vi "crio_RT_Radial_Antagonist_Closed_Loop_Vibration_Injection_with_Data_Logging.vi"() -> ()   [LabVIEW 2019]
uses:
  <vilib>/LabVIEW Targets/FPGA/cRIO/shared/nicrio_ModuleControls/nicrio_cRIO-9237_ExcitationVoltageRing.ctl
  <vilib>/Platform/TimedLoop/XDataNode/timing_clust.ctl
  <vilib>/Platform/TimedLoop/XDataNode/nitl_modes.ctl
  <vilib>/Platform/TimedLoop/XDataNode/wakeup.ctl
  <vilib>/FPGAPlugInAG/cRIO-9074/niLvFpga_Open_cRIO-9074.vi
  <vilib>/rvi/interface/common/dynamic/niFpgaDynamicAddResources.vi
  <vilib>/Utility/file.llb/Write Delimited Spreadsheet (string).vi
  <vilib>/Utility/error.llb/Error Cluster From Error Code.vi
  <vilib>/rvi/errors/niLvFpgaAdjustHostInterfaceError.vi
  <vilib>/Utility/file.llb/Write Delimited Spreadsheet (DBL).vi
  <vilib>/FPGAPlugInAG/Dynamic/niLvFpga_Close_Dynamic.vi
  <vilib>/rvi/interface/nirviOpenFPGA/nirviOpenFPGA.xnode
  On Call Bitfiles/gpass2_FPGATarget2_crioFPGAAntagoni_uWzRZvtrb5U.lvbitx
  <vilib>/rvi/interface/nirviReadWriteControl/nirviReadWriteControl.xnode
  <vilib>/platform/TimedLoop/XDataNode/XDataNode.xnode
  <vilib>/rvi/interface/nirviCloseFPGA/nirviCloseFPGA.xnode
  NiFpgaLv.dll
  <vilib>/rvi/interface/Simulation/niFpgaSimulationCallBeginRW.vi
  <vilib>/Platform/TimedLoop/XDataNode/XDNodeRunTimeDep.lvlib
panel:
  in  "LAC Gain Scaler":T1={"proportional gain"=100.0, "integral gain"=100000000.0}
  out "Trajectory time":dbl
  out "start time":timestamp
  out "LabVIEW TimeStamp":timestamp
  out "VCA Measured Position":i32=4
  out "LAC Setpoint":i32
  out "Rail Setpoint":i16
  out "VCA Setpoint":i32
  out "appended array":i32[](array[numeric])
  in  "Channel Names":string[](array[string])=["Channel 1", "Channel 2", "Channel 3", "Channel 4", "Channel 5"]
  in  "Header Info":string[][](array[string])=[["Test Name", "Operator", "UUT"], ["Voltage", "National Instruments", "AA123"]]
  out "error out":errorcluster
  out "log file path":path
  in  "precision test .csv name":string="precision_test.csv"
  in  "Default sin gain":dbl=20.0
  out "rail Platform Position":i16=4000
  out "LAC Measured Position":i32
  in  "VCA Loop Period(us)":i64=2000
  in  "VCA Position Reset":bool
  in  "VCA Velocity Interval (uSec)":u32=1000
  in  "LAC Position Reset":bool
  in  "LAC Velocity Interval (uSec)":u32=1000
  in  "LAC Lock":bool
  in  "Rail Manual Operation":bool
  in  "Rail Stepper Enable":bool
  in  "Rail Stepper Direction":bool
  in  "Half Peirod (pulse 40MHz)":u32=10000
  out "LAC Actual Gain":T1={"proportional gain"=0.009545455, "integral gain"=1.2626262e-09}
  in  "LAC manual control":T2={"manual? (F)"=FALSE, "manual input (0)"=-0.83838385} {"manual input (0)" scale=-1.0..1.0}
  in  "LAC setpoint":i32(slide)=2700 scale=0.0..4500.0
  in  "LAC Gains":T1={"proportional gain"=0.95454544, "integral gain"=0.64646465} {"proportional gain" scale=0.0..1.0; "integral gain" scale=0.0..1.0}
  in  "Rail Desired Position":i16(slide)=4000 scale=0.0..20000.0
  in  "PWM Frequency (default 20kHz)":i32=20000
  in  "Excitation Voltage":T3 items=["2.5 Volts", "3.3 Volts", "5.0 Volts", "10.0 Volts", "External Excitation"]
  out "scaled load cell reading":fxp<+/-,24,24>
  in  "VCA Manual Control":T2
  in  "VCA Gains":T1={"proportional gain"=0.25, "integral gain"=0.7979798} {"proportional gain" scale=0.0..1.0; "integral gain" scale=0.0..1.0}
  out "VCA Actual Gain":T1={"proportional gain"=0.0009797979, "integral gain"=7.979798e-09}
  in  "VCA Gain Scaler":T1={"proportional gain"=1000.0, "integral gain"=100000000.0}
  out "VCA Force Setpoint":sgl
  out "VCA Force":dbl(graph)
  out "PWM":sgl(graph)=0.061072454
  out "ControllerPWM Output":sgl=0.061072454
  out "ms to next point":u32=50500
  in  "Start Fequency":dbl=0.2
  out "Current Sweeping frequency":dbl=0.2
  in  "End Frequency":i32=20
  in  "Frequency Increment":dbl=1.0
  in  "Start Sweep":bool
  in  "Frequency":dbl=0.2
  in  "Lock_loop_rate":u32=5000
  in  "sin_gain":fxp<+,32,10>=0.25
  in  "sin_offset":fxp<+/-,32,10>=0.5
  in  "stop":bool
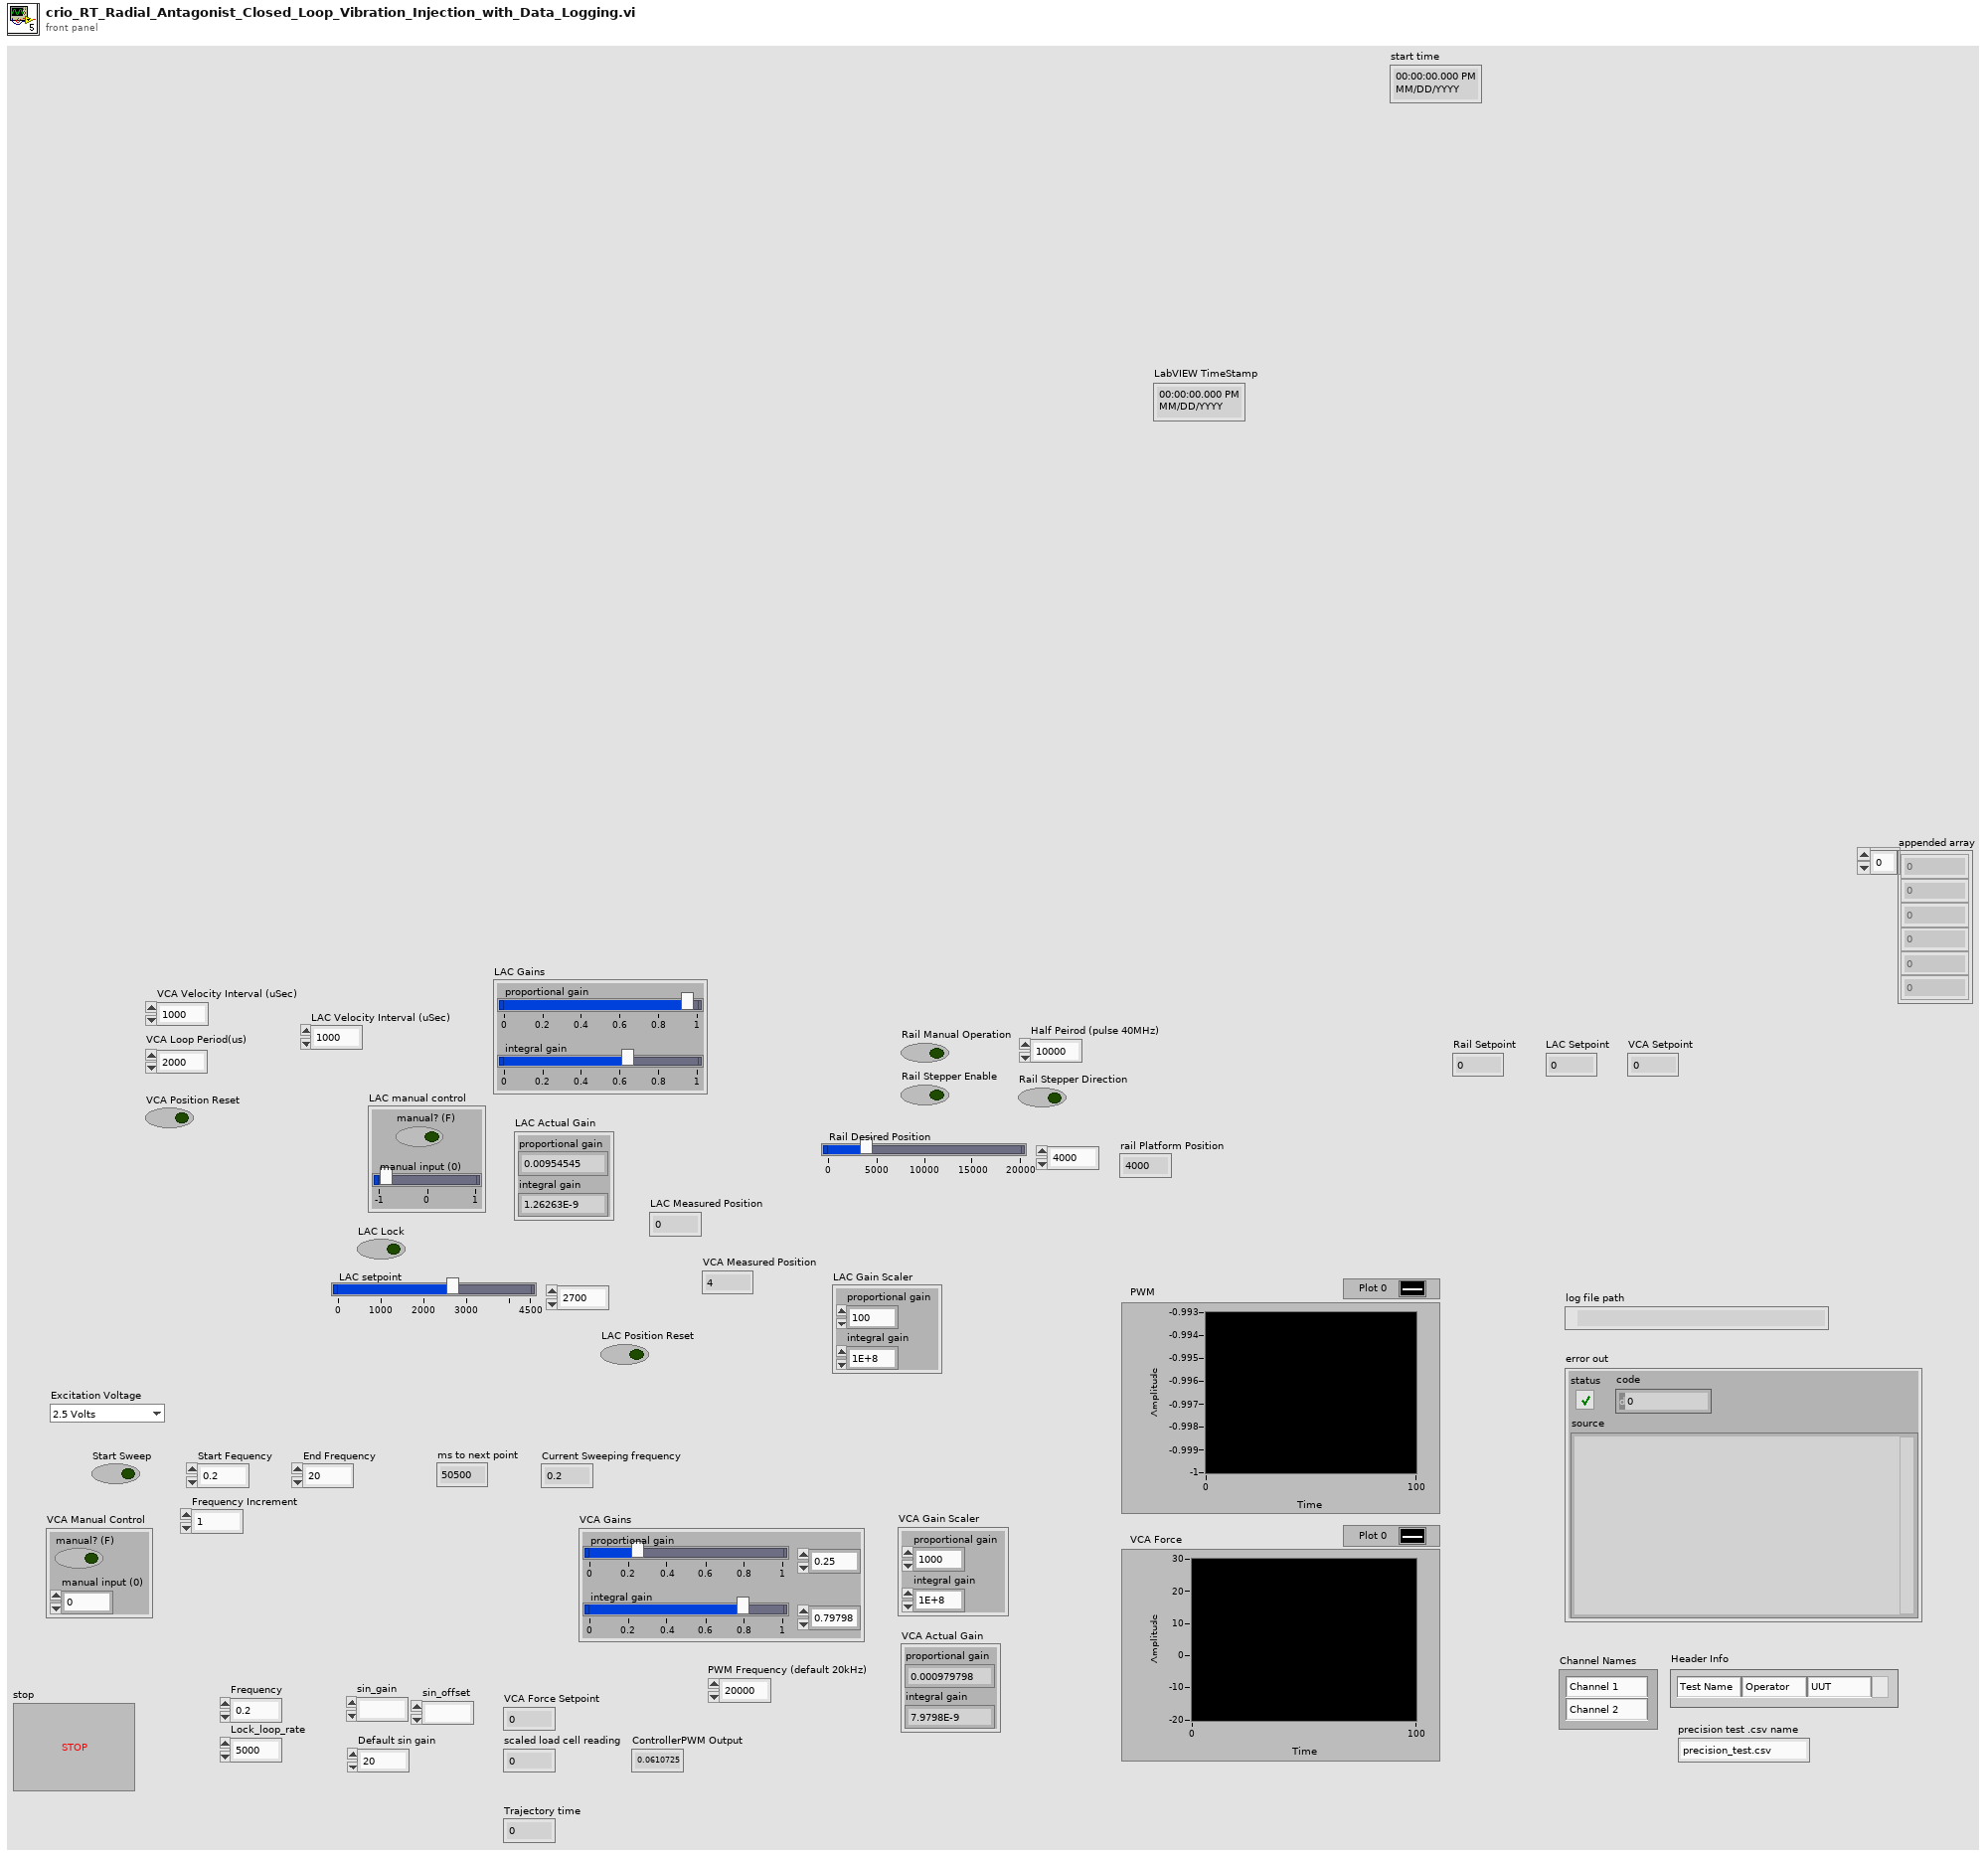
[diagram p1: front panel]
types:
  T1 = cluster{"proportional gain":sgl, "integral gain":sgl}
  T2 = cluster{"manual? (F)":bool, "manual input (0)":sgl}
  T3 = typedef "nicrio_cRIO-9237_ExcitationVoltageRing.ctl" = u8
  T4 = typedef "XDNodeRunTimeDep.lvlib/timing_clust.ctl" = cluster{"Expected End [f-1]":u64, "Actual End [f-1]":u64, "Finished Late? [f-1]":bool, "Expected End [i-1]":u64, "Actual End [i-1]":u64, "Finished Late? [i-1]":bool, "Expected Start [i]":u64, "Actual Start [i]":u64, "Expected Start [f]":u64, "Actual Start [f]":u64, "Source Name":string, "Structure Name":string, "Period":i64, "Deadline":i64, "Offset":i64, "Start":i64, "Priority":i32, "Timeout":i32, "Mode":T5, "Wakeup Reason":T6, "Error":errorcluster, "Source Type":string, "Secondary Source Type":string, "Global End Time":u64, "Global Start Time":u64, "Frame Duration":u64, "Iteration Duration":u64, "Assigned CPU":i32, "I/O Scan Engine Mode":u32}
  T5 = typedef "XDNodeRunTimeDep.lvlib/nitl_modes.ctl" = enum32{"No Change", "Process missed periods, maintain original phase", "Discard missed periods, maintain original phase", "Process missed periods, ignore original phase", "Discard missed periods, ignore original phase"}
  T6 = typedef "XDNodeRunTimeDep.lvlib/wakeup.ctl" = enum32{"Normal", "Aborted", "Asynchronous wakeup", "Timing source error", "Timed loop error", "Timeout"}
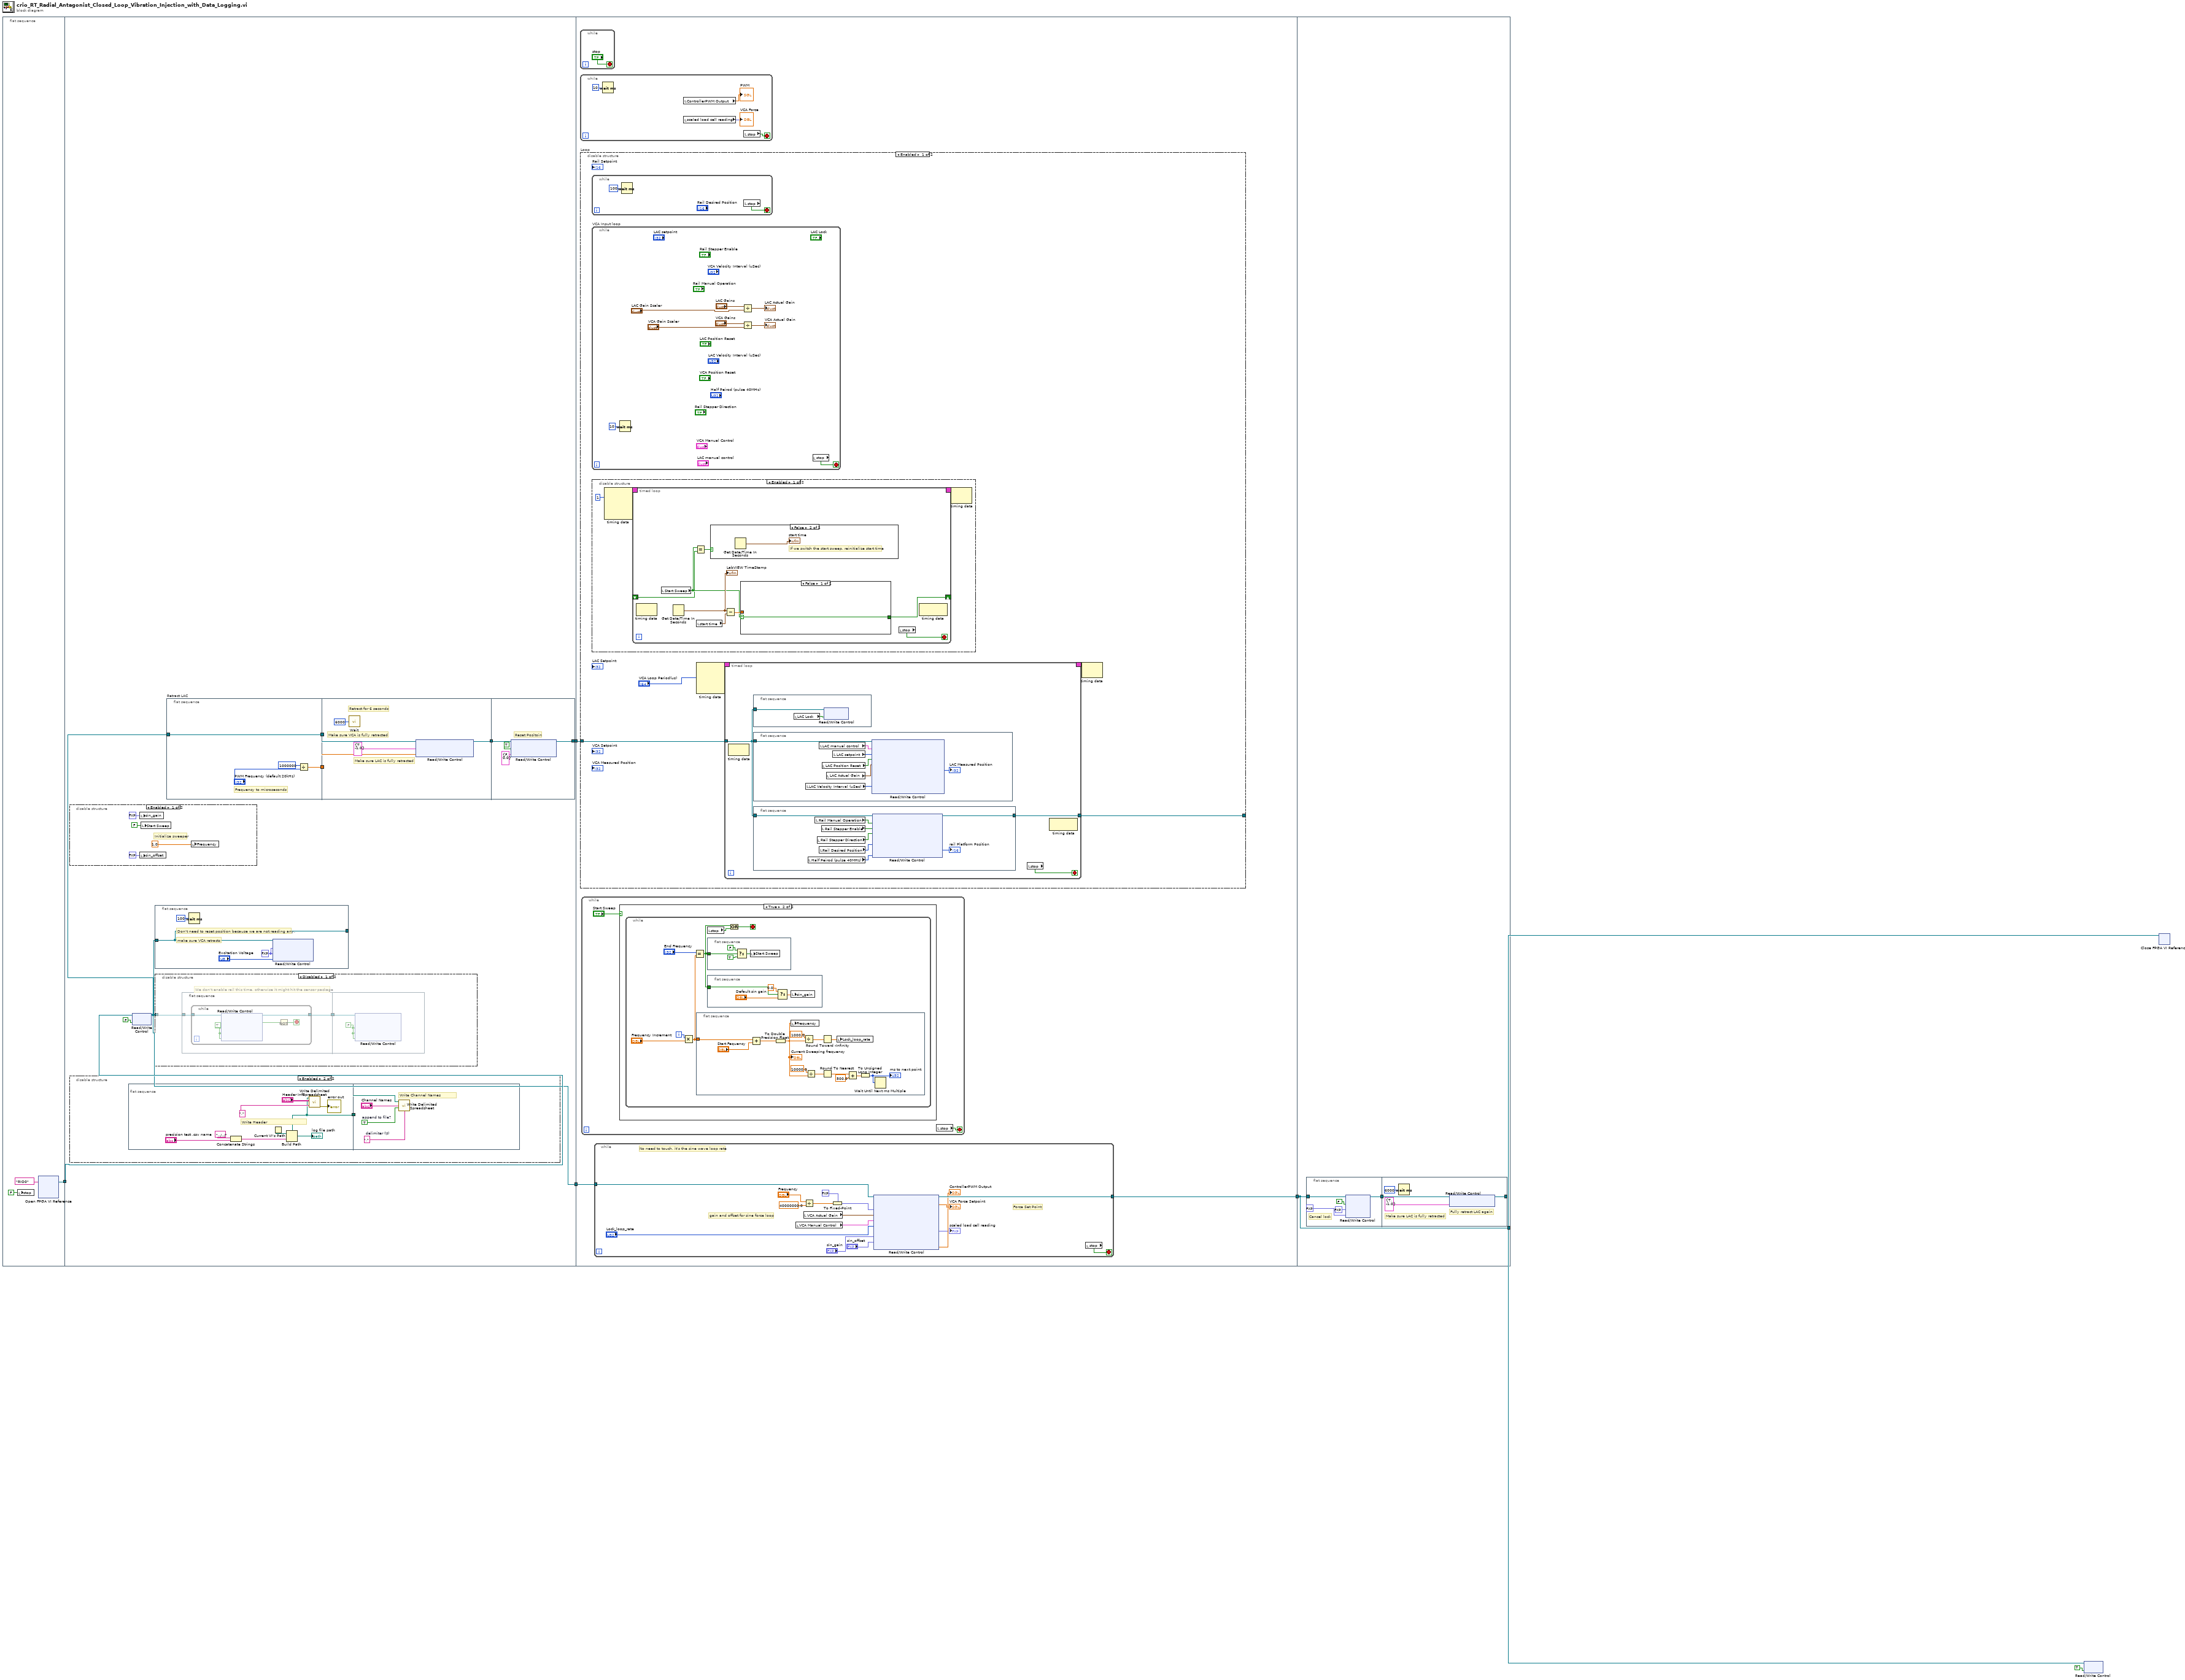
[diagram p0: block diagram]
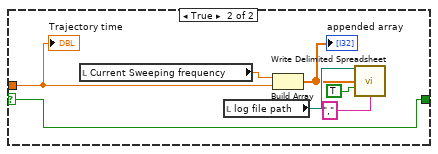
[diagram p6: hidden frame]
diagram:
  n1 = flat-sequence {
    tunnel: [w9] -> w6
    tunnel: w6 -> [w15]
    tunnel: [w11] -> w5
    tunnel: [w10] -> w3
    tunnel: w5 -> [w64]
    tunnel: [w63] -> w4
    tunnel: w3 -> [w62]
    tunnel: w4 -> [w183]
    tunnel: [w183] -> w1
    frame #0 {
      n2 = local write "stop"(FALSE ("stop")) -> ()
      n3 = xnode "Open FPGA VI Reference"("resource name"=tag "RIO0") -> ("FPGA VI Reference Out"=w9:refnum<k20>)  [unwired: 1 in, 1 out]
    }
    frame #1 {
      n4 = disable-structure shown="Enabled" {
        frame Enabled {
          # "Initialize sweeper"
          n5 = local write "sin_gain"(fxp<+,16,2> 0.0 ("sin_gain")) -> ()
          n6 = local write "sin_offset"(fxp<+/-,16,3> 0.0 ("sin_offset")) -> ()
          n7 = local write "Start Sweep"(FALSE ("Start Sweep")) -> ()
          n8 = local write "Frequency"(1.0 ("Frequency")) -> ()
        }
        frame Disabled {
        }
      }
      n9 = disable-structure shown="Enabled" {
        frame Disabled {
        }
        frame Enabled {
          n10 = flat-sequence {
            tunnel: [w21] -> w17
            tunnel: w17 -> [w26]
            frame #0 {
              # "Write Header"
              n11 = Concatenate Strings("../../" ("name or relative path"), "precision test .csv name") -> (w18:string)
              n12 = Current VI's Path() -> (path=w22:path)
              n13 = Build Path(base path=w22, name or relative path=w18) -> (appended path=w21:path)
              "log file path" <- w21
              n14 = call-poly <vilib>:"Write Delimited Spreadsheet.vi"("file path (dialog if empty)"=w21, "2D data"="Header Info", "delimiter (\\t)"="," ("delimiter (\\t)")) -> ("error out"=→"error out":errorcluster)  [unwired: 11 in, 1 out]
            }
            frame #1 {
              w28 = TRUE  # append to file?
              w27 = ","  # delimiter (\t)
              # "Write Channel Names"
              n15 = call-poly <vilib>:"Write Delimited Spreadsheet.vi"("file path (dialog if empty)"=w26, "1D data"="Channel Names", "append to file? (new file:F)"=w28, "delimiter (\\t)"=w27) -> ()  [unwired: 10 in, 2 out]
            }
          }
        }
      }
      n16 = xnode "Read/Write Control"("FPGA VI Reference In"=w15, "stop"=FALSE) -> ("FPGA VI Reference Out"=w11:refnum<k20>)  [unwired: 1 in, 1 out]
      n17 = flat-sequence {
        tunnel: [w58] -> _
        tunnel: w11 -> [w58]
        frame #0 {
          w61 = fxp<+/-,16,3> 0.0 ("sin_offset")
          # "Don't need to reset position because we are not reading any."
          # "make sure VCA retracts"
          n18 = Wait (ms)(milliseconds to wait=u32 100) -> ()  [unwired: 1 out]
          n19 = xnode "Read/Write Control"("FPGA VI Reference In"=w58, "sin_offset"=w61, "sin_gain"=w61, "Excitation Voltage"="Excitation Voltage") -> ()  [unwired: 1 in, 2 out]
        }
      }
      n20 = disable-structure shown="Disabled" {
        disable-tunnel: w11 -> [w47 _]
        frame Disabled {
          # "We don't enable rail this time, otherwise it might hit the sensor package"
          n21 = flat-sequence {
            tunnel: w47 -> [w49]
            tunnel: [w50] -> w48
            tunnel: w48 -> [w57]
            frame #0 {
              n22 = while {
                tunnel: [w54] -> w50
                tunnel: w49 -> [w53]
                stop <- w51 stop-if-true
                w55 = TRUE ("Stepper Direction")
                n23 = xnode "Read/Write Control"("FPGA VI Reference In"=w53, "Manual Operation"=w55, "Stepper Enable"=w55, "Stepper Direction"=w55) -> ("FPGA VI Reference Out"=w54:refnum<k20>, "Limit Switch"=w52:bool)  [unwired: 1 in, 1 out]
                n24 = Not(x=w52) -> (.not. x?=w51:bool)
              }
            }
            frame #1 {
              w56 = FALSE ("Stepper Direction")
              n25 = xnode "Read/Write Control"("FPGA VI Reference In"=w57, "Manual Operation"=w56, "Stepper Enable"=w56, "Stepper Direction"=w56) -> ()  [unwired: 1 in, 3 out]
            }
          }
        }
        frame Enabled {
          # "We don't enable rail this time, otherwise it might hit the sensor package"
        }
      }
      n26 = flat-sequence "Retract LAC" {
        tunnel: [w36] -> w14
        tunnel: w11 -> [w34]
        tunnel: [w34] -> w13
        tunnel: w14 -> [w41]
        tunnel: w13 -> [w39]
        tunnel: [w42] -> w12
        tunnel: w12 -> [w45]
        tunnel: [w46] -> w10
        frame #0 {
          # "Frequency to microseconds"
          n27 = Divide(x=1000000, y="PWM Frequency (default 20kHz)") -> (x/y=w36:dbl)
        }
        frame #1 {
          # "Make sure LAC is fully retracted"
          # "Retract for 6 seconds"
          # "Make sure VCA is fully retracted"
          n28 = call "Wait"("Count(mSec)"=u32 6000) -> ()  [unwired: 1 out]
          n29 = xnode "Read/Write Control"("FPGA VI Reference In"=w39, "LAC Manual Control"=T2 {"manual? (F)"=TRUE, "manual input (0)"=-1.0} ("manual control"), "DC PWM Period (microsec)"=w41) -> ("FPGA VI Reference Out"=w42:refnum<k20>)  [unwired: 1 in, 1 out]
        }
        frame #2 {
          # "Reset Positoin"
          n30 = xnode "Read/Write Control"("FPGA VI Reference In"=w45, "Position Reset"=TRUE, "LAC Manual Control"=T2 {"manual? (F)"=FALSE, "manual input (0)"=0.0} ("manual control")) -> ("FPGA VI Reference Out"=w46:refnum<k20>)  [unwired: 1 in, 1 out]
        }
      }
    }
    frame #2 {
      n31 = while {
        stop <- "stop" stop-if-true
      }
      n32 = while {
        stop <- w134 stop-if-true
        n33 = Wait (ms)(milliseconds to wait=u32 10) -> ()  [unwired: 1 out]
        n34 = local read "ControllerPWM Output"() -> (→"PWM":sgl)
        n35 = local read "scaled load cell reading"() -> (→"VCA Force":fxp<+/-,24,24>)
        n36 = local read "stop"() -> (w134:bool)
      }
      n37 = disable-structure "Loop" shown="Enabled" {
        disable-tunnel: w62 -> [w66 _]
        disable-tunnel: [w65 _] -> _
        frame Enabled {
          n38 = while {
            stop <- w96 stop-if-true
            n39 = Wait (ms)(milliseconds to wait=u32 100) -> ()  [unwired: 1 out]
            n40 = local read "stop"() -> (w96:bool)
          }
          n41 = while "VCA Input loop" {
            stop <- w104 stop-if-true
            n42 = Wait (ms)(milliseconds to wait=u32 10) -> ()  [unwired: 1 out]
            n43 = Divide(x="LAC Gains", y="LAC Gain Scaler") -> (x/y=→"LAC Actual Gain":T1)
            n44 = Divide(x="VCA Gains", y="VCA Gain Scaler") -> (x/y=→"VCA Actual Gain":T1)
            n45 = local read "stop"() -> (w104:bool)
          }
          n46 = disable-structure shown="Enabled" {
            frame Enabled {
              n47 = node-c288(i64 1 ("Period")) -> (w72:T4)  [unwired: 3 in]
              n48 = timed-loop {
                timing: w72 -> [_]
                timing-out: [_] -> w71
                shift-right: [w76] -> _
                shift-left: _ -> [w74]
                stop <- w80 stop-if-true
                n49 = node-c288() -> ()  [unwired: 1 in, 1 out]
                n50 = local read "Start Sweep"() -> (w75:bool)
                n51 = Get Date/Time In Seconds() -> (seconds since 1Jan1904=w78:timestamp)
                "LabVIEW TimeStamp" <- w78
                n52 = Equal?(x=w75, y=w74) -> (x = y?=w73:bool)
                n53 = local read "start time"() -> (w79:timestamp)
                n54 = case shown="False" w73 {
                  frame True {
                  }
                  frame False {
                    # "If we switch the start sweep, reinitialize start time"
                    n55 = Get Date/Time In Seconds() -> (seconds since 1Jan1904=→"start time":timestamp)
                  }
                }
                n56 = Subtract(x=w78, y=w79) -> (x-y=w77:dbl)
                n57 = case shown="False" w75 {
                  selector: w75 -> [w82 w83]
                  tunnel: w77 -> [_ w84]
                  tunnel: [w82 w83] -> w76
                  frame False {
                  }
                  frame True {
                    n58 = local read "Current Sweeping frequency"() -> (w85:dbl)
                    n59 = local read "log file path"() -> (w89:path)
                    n60 = Build Array(w85, w84) -> (w88:dbl[])
                    "appended array" <- w88
                    n61 = call-poly <vilib>:"Write Delimited Spreadsheet.vi"("file path (dialog if empty)"=w89, "1D data"=w88, "append to file? (new file:F)"=TRUE, "delimiter (\\t)"="," ("delimiter (\\t)")) -> ()  [unwired: 10 in, 2 out]
                    "Trajectory time" <- w84
                  }
                }
                n62 = local read "stop"() -> (w80:bool)
                n63 = node-c288() -> ()  [unwired: 1 in, 1 out]
              }
              n64 = node-c288(w71) -> ()  [unwired: 1 out]
            }
            frame Disabled {
            }
          }
          n65 = node-c288("VCA Loop Period(us)") -> (w69:T4)  [unwired: 3 in]
          n66 = timed-loop {
            timing: w69 -> [_]
            timing-out: [_] -> w68
            tunnel: w66 -> [w106]
            tunnel: [w107] -> w65
            stop <- w108 stop-if-true
            n67 = node-c288() -> ()  [unwired: 1 in, 1 out]
            n68 = flat-sequence {
              tunnel: w106 -> [w125]
              frame #0 {
                n69 = local read "LAC Lock"() -> (w124:bool)
                n70 = xnode "Read/Write Control"("FPGA VI Reference In"=w125, "LAC Lock"=w124) -> ()  [unwired: 1 in, 2 out]
              }
            }
            n71 = flat-sequence {
              tunnel: w106 -> [w115]
              frame #0 {
                n72 = local read "LAC Velocity Interval (uSec)"() -> (w110:u32)
                n73 = local read "LAC manual control"() -> (w114:T2)
                n74 = local read "LAC Position Reset"() -> (w112:bool)
                n75 = local read "LAC Actual Gain"() -> (w111:T1)
                n76 = local read "LAC setpoint"() -> (w113:i32)
                n77 = xnode "Read/Write Control"("FPGA VI Reference In"=w115, "LAC Manual Control"=w114, "LAC Setpoint"=w113, "Position Reset"=w112, "LAC Gains"=w111, "LAC Velocity Interval (uSec)"=w110) -> ("LAC Position (Counts)"=→"LAC Measured Position":i32)  [unwired: 1 in, 5 out]
              }
            }
            n78 = flat-sequence {
              tunnel: w106 -> [w117]
              tunnel: [w116] -> w107
              frame #0 {
                n79 = local read "Half Peirod (pulse 40MHz)"() -> (w123:u32)
                n80 = local read "Rail Manual Operation"() -> (w119:bool)
                n81 = local read "Rail Stepper Direction"() -> (w120:bool)
                n82 = local read "Rail Desired Position"() -> (w122:i16)
                n83 = local read "Rail Stepper Enable"() -> (w121:bool)
                n84 = xnode "Read/Write Control"("FPGA VI Reference In"=w117, "Manual Operation"=w119, "Stepper Enable"=w121, "Stepper Direction"=w120, "Position Control: Desired Positoin"=w122, "Half Peirod (pulse 40MHz)"=w123) -> ("FPGA VI Reference Out"=w116:refnum<k20>, "rail Platform Position"=→"rail Platform Position":i16)  [unwired: 2 in, 1 out]
              }
            }
            n85 = local read "stop"() -> (w108:bool)
            n86 = node-c288() -> ()  [unwired: 1 in, 1 out]
          }
          n87 = node-c288(w68) -> ()  [unwired: 1 out]
        }
        frame Disabled {
        }
      }
      n88 = while {
        stop <- w137 stop-if-true
        n89 = case shown="True" "Start Sweep" {
          frame False {
          }
          frame True {
            n90 = while {
              i -> [w141]
              stop <- w144 stop-if-true
              n91 = Multiply(x=w141, y="Frequency Increment") -> (x*y=w140:dbl)
              n92 = Equal?(x="End Frequency", y=w140) -> (x = y?=w138:bool)
              n93 = flat-sequence {
                tunnel: w140 -> [w158]
                frame #0 {
                  n94 = Add(x=w158, y="Start Fequency") -> (x+y=w159:dbl)
                  n95 = To Double Precision Float(number=w159) -> (double precision float=w153:dbl)
                  "Current Sweeping frequency" <- w153
                  n96 = local write "Frequency"(w153) -> ()
                  n97 = Divide(x=1000.0 ("y"), y=w153) -> (x/y=w156:dbl)
                  n98 = Divide(x=10000.0 ("y"), y=w153) -> (x/y=w165:dbl)
                  n99 = Round Toward -Infinity(1:w156) -> (0:w155:dbl)
                  n100 = Round To Nearest(number=w165) -> (nearest integer value=w162:dbl)
                  n101 = local write "Lock_loop_rate"(w155) -> ()
                  n102 = Add(x=w162, y=500.0) -> (x+y=w160:dbl)
                  n103 = To Unsigned Long Integer(number=w160) -> (unsigned 32bit integer=w163:u32)
                  "ms to next point" <- w163
                  n104 = Wait Until Next ms Multiple(millisecond multiple=w163) -> ()  [unwired: 1 out]
                }
              }
              n105 = local read "stop"() -> (w143:bool)
              n106 = flat-sequence {
                tunnel: w138 -> [w152]
                frame #0 {
                  n107 = Select(t=FALSE, s=w152, f=TRUE) -> (s? t:f=w150:bool)
                  n108 = local write "Start Sweep"(w150) -> ()
                }
              }
              n109 = flat-sequence {
                tunnel: w138 -> [w148]
                frame #0 {
                  n110 = Select(t=0.0, s=w148, f="Default sin gain") -> (s? t:f=w147:dbl)
                  n111 = local write "sin_gain"(w147) -> ()
                }
              }
              n112 = Or(x=w138, y=w143) -> (x .or. y?=w144:bool)
            }
          }
        }
        n113 = local read "stop"() -> (w137:bool)
      }
      n114 = while {
        tunnel: w64 -> [w180]
        tunnel: [w171] -> w63
        stop <- w181 stop-if-true
        # "Force Set Point"
        # "gain and offset for sine force loop"
        # "No need to touch, it's the sine wave loop rate"
        n115 = local read "VCA Manual Control"() -> (w167:T2)
        n116 = local read "VCA Actual Gain"() -> (w168:T1)
        n117 = Divide(x="Frequency", y=40000000.0) -> (x/y=w178:dbl)
        n118 = To Fixed-Point(fixed-point type=fxp<+,32,0> 0.0 ("frequency (periods/tick)"), number=w178) -> (fixed-point=w175:fxp<+,32,0>)
        n119 = xnode "Read/Write Control"("FPGA VI Reference In"=w180, "sweep frequency (periods/tick)"=w175, "VCA Gains"=w168, "VCA Manual Control"=w167, "Lock_loop_rate"="Lock_loop_rate", "sin_gain"="sin_gain", "sin_offset"="sin_offset") -> ("FPGA VI Reference Out"=w171:refnum<k20>, "VCA Force Setpoint"=→"VCA Force Setpoint":sgl, "scaled load cell reading"=→"scaled load cell reading":fxp<+/-,24,24>, "VCA ControllerPWM Output"=→"ControllerPWM Output":sgl)  [unwired: 1 in, 1 out]
        n120 = local read "stop"() -> (w181:bool)
      }
    }
    frame #3 {
      n121 = flat-sequence {
        tunnel: w183 -> [w189]
        tunnel: [w188] -> w184
        tunnel: [w192] -> _
        tunnel: w184 -> [w193]
        frame #0 {
          # "Cancel lock"
          n122 = xnode "Read/Write Control"("FPGA VI Reference In"=w189, "LAC Lock"=FALSE, "sin_offset"=fxp<+/-,16,3> -1.0, "sin_gain"=fxp<+,32,1> 0.0) -> ("FPGA VI Reference Out"=w188:refnum<k20>)  [unwired: 1 in, 1 out]
        }
        frame #1 {
          # "Make sure LAC is fully retracted"
          # "Fully retract LAC again"
          n123 = Wait (ms)(milliseconds to wait=u32 6000) -> ()  [unwired: 1 out]
          n124 = xnode "Read/Write Control"("FPGA VI Reference In"=w193, "LAC Manual Control"=T2 {"manual? (F)"=TRUE, "manual input (0)"=-1.0} ("manual control")) -> ("FPGA VI Reference Out"=w192:refnum<k20>)  [unwired: 1 in, 1 out]
        }
      }
    }
  }
  n125 = xnode "Read/Write Control"("FPGA VI Reference In"=w1, "stop"=TRUE) -> ()  [unwired: 1 in, 2 out]
  n126 = xnode "Close FPGA VI Reference"("FPGA VI Reference In"=w1) -> ()  [unwired: 1 in, 1 out]
